vi "To String (Null).vi"(8 "error in (no error)":errorcluster) -> (0 "error out":errorcluster, 3 "String":string)   [LabVIEW 2017, in "Advanced Variant Tools.lvlib"]
doc: "Flattens the given JSON data to a string."
uses:
  Advanced Variant Tools.lvlib
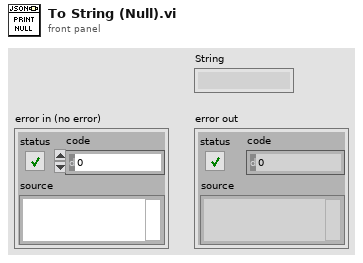
[diagram p1: front panel]
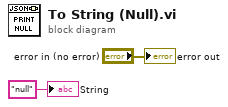
[diagram p0: block diagram]
diagram:
  "String" <- "null" ("String")
  "error out" <- "error in (no error)"
